vi "Judge API Plan.vi"(11 "DeepL authKey":string) -> (3 "DeepL Free API?":bool)   [LabVIEW 2015, in "lv-deepl-api.lvlib"]
uses:
  lv-deepl-api.lvlib
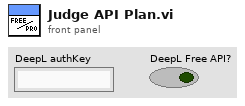
[diagram p1: front panel]
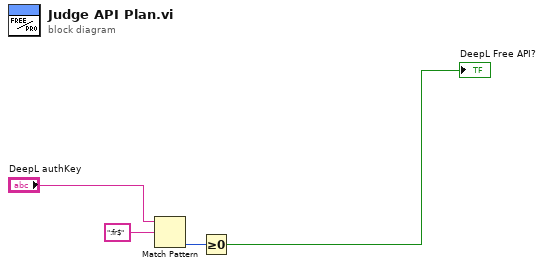
[diagram p0: block diagram]
diagram:
  n1 = Match Pattern(string="DeepL authKey", regular expression=":fr$" ("正規表現")) -> (offset past match=w3:i32)  [unwired: 1 in, 3 out]
  n2 = Greater Or Equal To 0?(x=w3) -> (x >= 0?=→"DeepL Free API?":bool)
